vi "Find Direction.vi"(10 "Src":cluster{i32, "index of element":i32}, 11 "Dest":cluster{i32, "index of element":i32}) -> (3 "Dir":string)   [LabVIEW 2023, in "d10.lvlib"]
uses:
  d10.lvlib
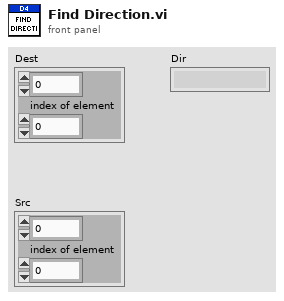
[diagram p1: front panel]
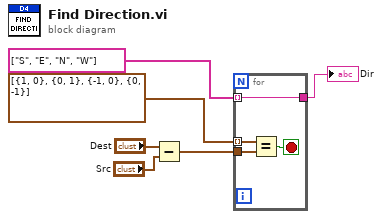
[diagram p0: block diagram]
diagram:
  n1 = Subtract(x="Dest", y="Src") -> (x-y=w5:cluster{i32, "index of element":i32})
  n2 = for {
    tunnel: w5 -> [w10]
    tunnel: cluster{i32, i32}[] [{1, 0}, {0, 1}, {-1, 0}, {0, -1}] -> [w9] mode=indexing
    tunnel: string[] ["S", "E", "N", "W"] -> [w7] mode=indexing
    tunnel: [w7] -> w6
    stop <- w8 stop-if-true
    n3 = Equal?(x=w9, y=w10) -> (x = y?=w8:bool)
  }
  "Dir" <- w6
